vi "Selection Indices.vi"(8 "error in (no error)":errorcluster, 10 "Channel Tree Tag":string, 11 "GenericGuiAO in":refnum<class "GenericGuiDO.lvclass">) -> (0 "error out":errorcluster, 3 "GenericGuiAO out":refnum<class "GenericGuiDO.lvclass">)   [LabVIEW 2020, in "VolatusDAQGenericGUI.lvlib" / "GenericGuiDO.lvclass"]
uses:
  GenericGuiDO.lvclass
  GenericGuiDO.lvclass/GenericGuiDO.ctl
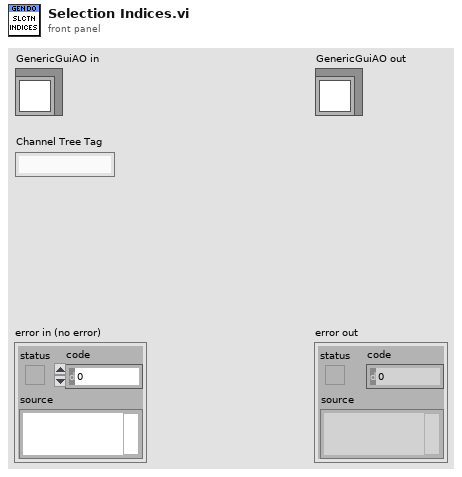
[diagram p1: front panel]
types:
  T1 = typedef "VolatusDAQGenericGUI.lvlib/Group Info.ctl" = cluster{"Group":refnum<class "Group.lvclass">, "Channel Names":string[], "Resources":string[], "Node":string, "Task":string}
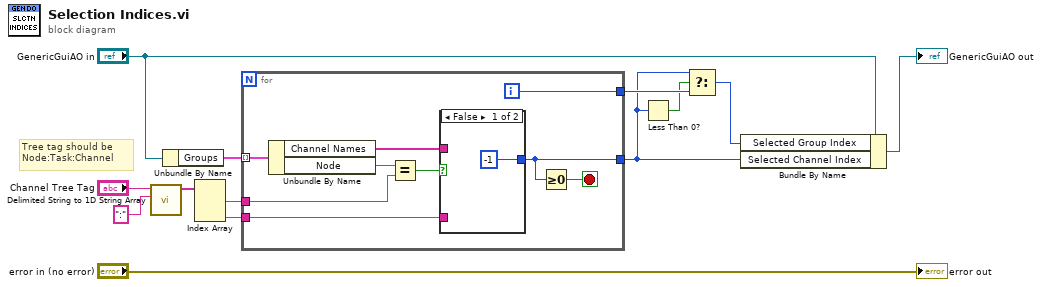
[diagram p0: block diagram]
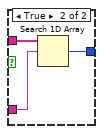
[diagram p2: hidden frame]
diagram:
  # "Tree tag should be\nNode:Task:Channel"
  n1 = call <vilib>:"Delimited String to 1D String Array.vi"("delimiter"=":", "delimited string"="Channel Tree Tag") -> ("string array"=w8:string[])  [unwired: 9 in]
  n2 = Unbundle By Name("GenericGuiAO in") -> ("Groups"=w9:T1[])
  n3 = Index Array(array=w8) -> (element #1=w7:string, element #3=w6:string)  [unwired: 3 in, 1 out]
  n4 = for {
    tunnel: w9 -> [w22] mode=indexing
    tunnel: w7 -> [w20]
    tunnel: w6 -> [w17]
    tunnel: [w16] -> w4
    tunnel: [w15] -> w2
    i -> [w16]
    stop <- w14 stop-if-true
    n5 = Unbundle By Name(w22) -> ("Channel Names"=w18:string[], "Node"=w21:string)
    n6 = Equal?(x=w21, y=w20) -> (x = y?=w19:bool)
    n7 = case shown="False" w19 {
      tunnel: w18 -> [_ w26]
      tunnel: w17 -> [_ w25]
      tunnel: [-1 ("index of element") w24] -> w15
      frame False {
      }
      frame True {
        n8 = Search 1D Array(1D array=w26, element=w25) -> (index of element=w24:i32)  [unwired: 1 in]
      }
    }
    n9 = Greater Or Equal To 0?(x=w15) -> (x >= 0?=w14:bool)
  }
  n10 = Less Than 0?(x=w2) -> (x < 0?=w3:bool)
  n11 = Select(t=w2, s=w3, f=w4) -> (s? t:f=w1:i32)
  n12 = Bundle By Name(cluster="GenericGuiAO in", "Selected Group Index"=w1, "Selected Channel Index"=w2) -> (→"GenericGuiAO out":refnum<class "GenericGuiDO.lvclass">)
  "error out" <- "error in (no error)"
